vi "Default Doc Settings Path.vi"() -> (3 "Default Doc Settings Path":path)   [LabVIEW 2023]
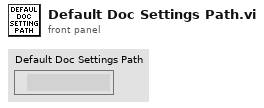
[diagram p1: front panel]
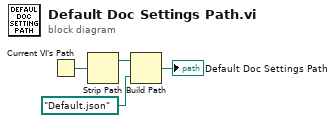
[diagram p0: block diagram]
diagram:
  n1 = Current VI's Path() -> (path=w3:path)
  n2 = Strip Path(path=w3) -> (stripped path=w2:path)  [unwired: 1 out]
  n3 = Build Path(base path=w2, name or relative path=path "Default.json") -> (appended path=→"Default Doc Settings Path":path)
